vi "Scripting_FollowWireToInnerTerm.vi"(0 "Term Refnum":refnum<vi>, 5 "error in":errorcluster) -> (14 "reference":refnum<vi>, 19 "error out":errorcluster)   [LabVIEW 2016]
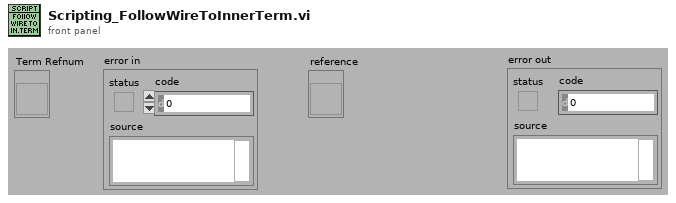
[diagram p1: front panel]
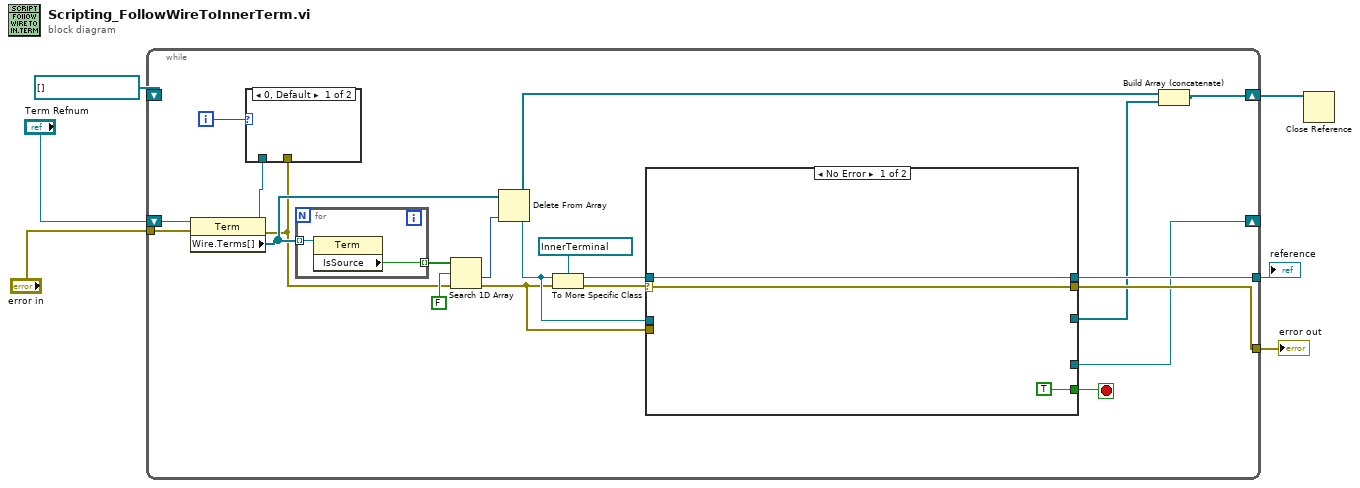
[diagram p0: block diagram]
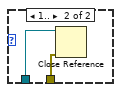
[diagram p2: hidden frame]
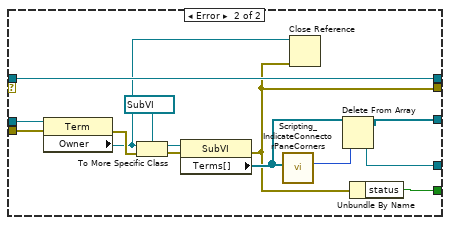
[diagram p3: hidden frame]
diagram:
  n1 = while {
    tunnel: "error in" -> [w22]
    tunnel: [w19] -> w4
    tunnel: [w18] -> w3
    shift-right: [w16] -> w1
    shift-left: refnum<vi>[] [] -> [_]
    shift-right: [w15] -> _
    shift-left: "Term Refnum" -> [w25]
    i -> [w7]
    stop <- w14 stop-if-true
    n2 = property class="Term"(reference=w25, error in=w22) -> (reference out=w8:refnum<vi>, error out=w9:errorcluster, "Wire.Terms[]"=w12:refnum<vi>[])
    n3 = case shown="0, Default" w7 {
      tunnel: w9 -> [_ w28]
      tunnel: w8 -> [_ w27]
      frame 0, Default {
      }
      frame 1.. {
        n4 = Close Reference(reference=w27, error in (no error)=w28) -> ()  [unwired: 1 out]
      }
    }
    n5 = for {
      tunnel: w12 -> [w47] mode=indexing
      tunnel: [w46] -> w24 mode=indexing
      n6 = property class="Term"(reference=w47) -> ("IsSource"=w46:bool)  [unwired: 1 in, 2 out]
    }
    n7 = Search 1D Array(1D array=w24, element=FALSE) -> (index of element=w13:i32)  [unwired: 1 in]
    n8 = Delete From Array(array=w12, index=w13) -> (deleted portion=w10:refnum<vi>, array with subset deleted=w11:refnum<vi>[])  [unwired: 1 in]
    n9 = To More Specific Class(target class=refnum<vi> refnum ("reference"), reference=w10, error in=w9) -> (specific class reference=w20:refnum<vi>, error out=w21:errorcluster)
    n10 = case shown="No Error" w21 {
      selector: w21 -> [w30 _]
      tunnel: w20 -> [w31 w43]
      tunnel: [w31 w43] -> w19
      tunnel: [w30 w33] -> w18
      tunnel: w10 -> [_ w45]
      tunnel: w9 -> [_ w44]
      tunnel: [_ w36] -> w17
      tunnel: [_ w34] -> w15
      tunnel: [TRUE ("status") w38] -> w14
      frame No Error {
      }
      frame Error {
        n11 = property class="Term"(reference=w45, error in=w44) -> (error out=w41:errorcluster, "Owner"=w32:refnum<vi>)  [unwired: 1 out]
        n12 = To More Specific Class(target class=refnum<vi> refnum ("reference"), reference=w32, error in=w41) -> (specific class reference=w40:refnum<vi>, error out=w39:errorcluster)
        n13 = property class="SubVI"(reference=w40, error in=w39) -> (error out=w33:errorcluster, "Terms[]"=w37:refnum<vi>[])  [unwired: 1 out]
        n14 = call <resource>:"Scripting_IndicateConnectorPaneCorners.vi"("Terminals[]"=w37) -> ("RightTop"=w35:i32)  [unwired: 7 in, 3 out]
        n15 = Close Reference(reference=w32, error in (no error)=w33) -> ()  [unwired: 1 out]
        n16 = Delete From Array(array=w37, index=w35) -> (deleted portion=w34:refnum<vi>, array with subset deleted=w36:refnum<vi>[])  [unwired: 1 in]
        n17 = Unbundle By Name(w33) -> ("status"=w38:bool)
      }
    }
    n18 = Build Array (concatenate)(w11, w17) -> (w16:refnum<vi>[])
  }
  "error out" <- w3
  "reference" <- w4
  n19 = Close Reference(reference=w1) -> ()  [unwired: 1 in, 1 out]
